vi "线性放大.vi"() -> ()   [LabVIEW 2018]
uses:
  <vilib>/measure/NI_MABase.lvlib
panel:
  in  "放大偏移量":dbl
  in  "停止":bool
  in  "放大系数":dbl
  out "波形图 2":waveform(dbl)(graph)
  out "波形图":waveform(dbl)(graph)
  in  "offset":dbl caption="原始信号偏移量" format="%0.2p"
  in  "sampling info":cluster{"Fs":dbl, "#s":dbl}={"Fs"=1000.0, "#s"=1000.0} caption="采样信息" {"Fs" format="%.2p"}
  in  "amplitude":dbl=1.0 caption="幅值" format="%0.2p"
  in  "frequency":dbl=10.0 caption="频率" format="%0.2p"
  in  "signal type":T1(ring) caption="信号类型"
  out "字符串":string="线性放大：y=kx+c"
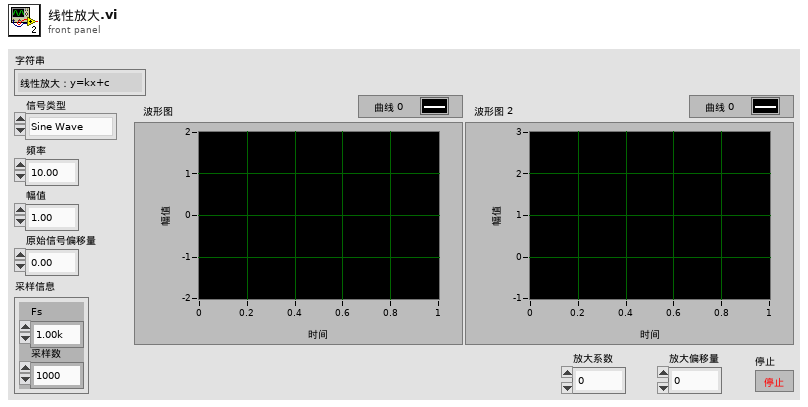
[diagram p1: front panel]
types:
  T1 = enum16{"Sine Wave", "Triangle Wave", "Square Wave", "Sawtooth Wave"}
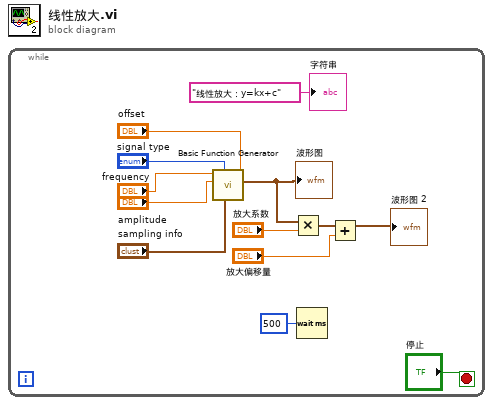
[diagram p0: block diagram]
diagram:
  n1 = while {
    stop <- "停止" stop-if-true
    n2 = call <vilib>:"Basic Function Generator.vi"("offset"="offset", "sampling info"="sampling info", "signal type"="signal type", "amplitude"="amplitude", "frequency"="frequency") -> ("signal out"=w7:waveform(dbl))  [unwired: 4 in, 2 out]
    "波形图" <- w7
    n3 = Multiply(x=w7, y="放大系数") -> (x*y=w5:waveform(dbl))
    n4 = Wait (ms)(milliseconds to wait=u32 500 ("等待时间（毫秒）")) -> ()  [unwired: 1 out]
    n5 = Add(x=w5, y="放大偏移量") -> (x+y=→"波形图 2":waveform(dbl))
    "字符串" <- "线性放大：y=kx+c"
  }
